vi "writeToXML.vi"(8 "error in (no error)":errorcluster, 10 "ClassLabel":string, 11 "M1Cover in":refnum<class "M1Cover.lvclass">) -> (0 "error out":errorcluster, 2 "XML out":string, 3 "M1Cover out":refnum<class "M1Cover.lvclass">)   [LabVIEW 2022 SP3, in "TCSDataDefinitions.lvlib" / "TCSCommand.lvlib" / "M1Cover.lvclass"]
uses:
  M1Cover.lvclass
  M1Cover.lvclass/M1Cover.ctl
  TCSTcsCommand/TCSTcsCommand.lvclass
  <userlib>/Common/XML/XMLGenerator/XMLGenerator.lvclass
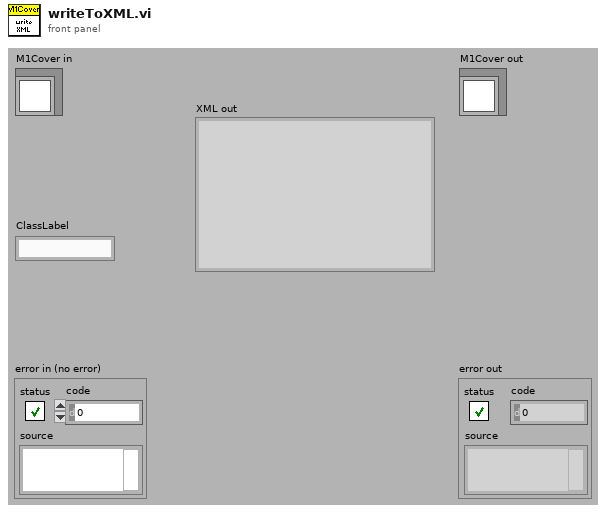
[diagram p1: front panel]
types:
  T1 = typedef "TCSDataDefinitions.lvlib/TCSCommand.lvlib/M1CoverMoveTypes.ctl" = enum16{"open", "close", "stop"}
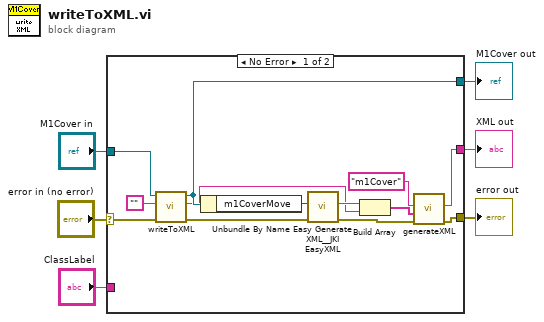
[diagram p0: block diagram]
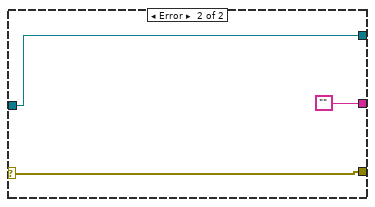
[diagram p2: hidden frame]
diagram:
  n1 = case shown="No Error" "error in (no error)" {
    selector: "error in (no error)" -> [w8 w22]
    tunnel: [w15 w22] -> w5
    tunnel: [w12 w21] -> w3
    tunnel: "M1Cover in" -> [w13 w21]
    tunnel: "ClassLabel" -> [_ _]
    tunnel: [w14 ""] -> w1
    frame No Error {
      n2 = call-parent "writeToXML.vi"("error in (no error)"=w8, "ClassLabel"="", "TCSTcsCommand in"=w13) -> ("error out"=w7:errorcluster, "XML out"=w10:string, "TCSTcsCommand out"=w12:refnum<class "M1Cover.lvclass">)  [unwired: 6 in]
      n3 = Unbundle By Name(w12) -> ("m1CoverMove"=w19:T1)
      n4 = call <vilib>:"Easy Generate XML__JKI EasyXML.vi"("error in (no error)"=w7, "LabVIEW Data"=w19) -> ("error out"=w16:errorcluster, "XML String"=w17:string)  [unwired: 8 in]
      n5 = Build Array(w17, w10) -> (w18:string[])
      n6 = call <userlib>:"generateXML.vi"("error in"=w16, "childrenXML"=w18, "elementName"="m1Cover" ("Class Label")) -> ("error out"=w15:errorcluster, "XML out"=w14:string)  [unwired: 6 in, 1 out]
    }
    frame Error {
    }
  }
  "error out" <- w5
  "M1Cover out" <- w3
  "XML out" <- w1
